vi "ConfigurationSetting_Dialog.vi"(2 "error in (no error)":errorcluster, 3 "Configuration":refnum<vi>) -> (0 "error out":errorcluster, 1 "Cancelled?":bool)   [LabVIEW 2012]
doc: "Use this template to create a dialog box with event handling."
uses:
  Config.ctl
panel:
  in  "Unblock":bool
  in  "Background WL":dbl=275.0 min=1.0 max=320.0
  in  "Knee Max":dbl min=0.0 max=40.0
  in  "Knee Min":dbl min=-40.0 max=0.0
  in  "Power Min":dbl min=0.0 max=10000.0
  in  "# Samples":i32=1 min=1 max=10
  in  "Int Time":i32=10 min=10 max=100000
  in  "Cancel":bool
  in  "Save":bool
  # "Configuration Settings"
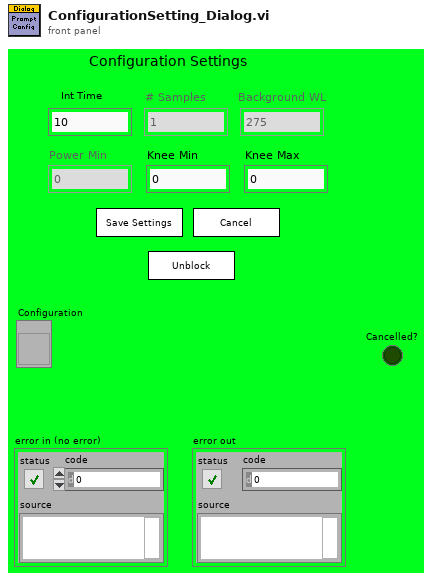
[diagram p1: front panel]
types:
  T1 = enum8{"Enabled", "Disabled", "Disabled and Grayed Out"}
  T2 = typedef "Config.ctl" = cluster{"IntTime":i32, "Samples":i32, "PowerMin":dbl, "KneeMin":dbl, "KneeMax":dbl, "BackgroundWl":dbl}
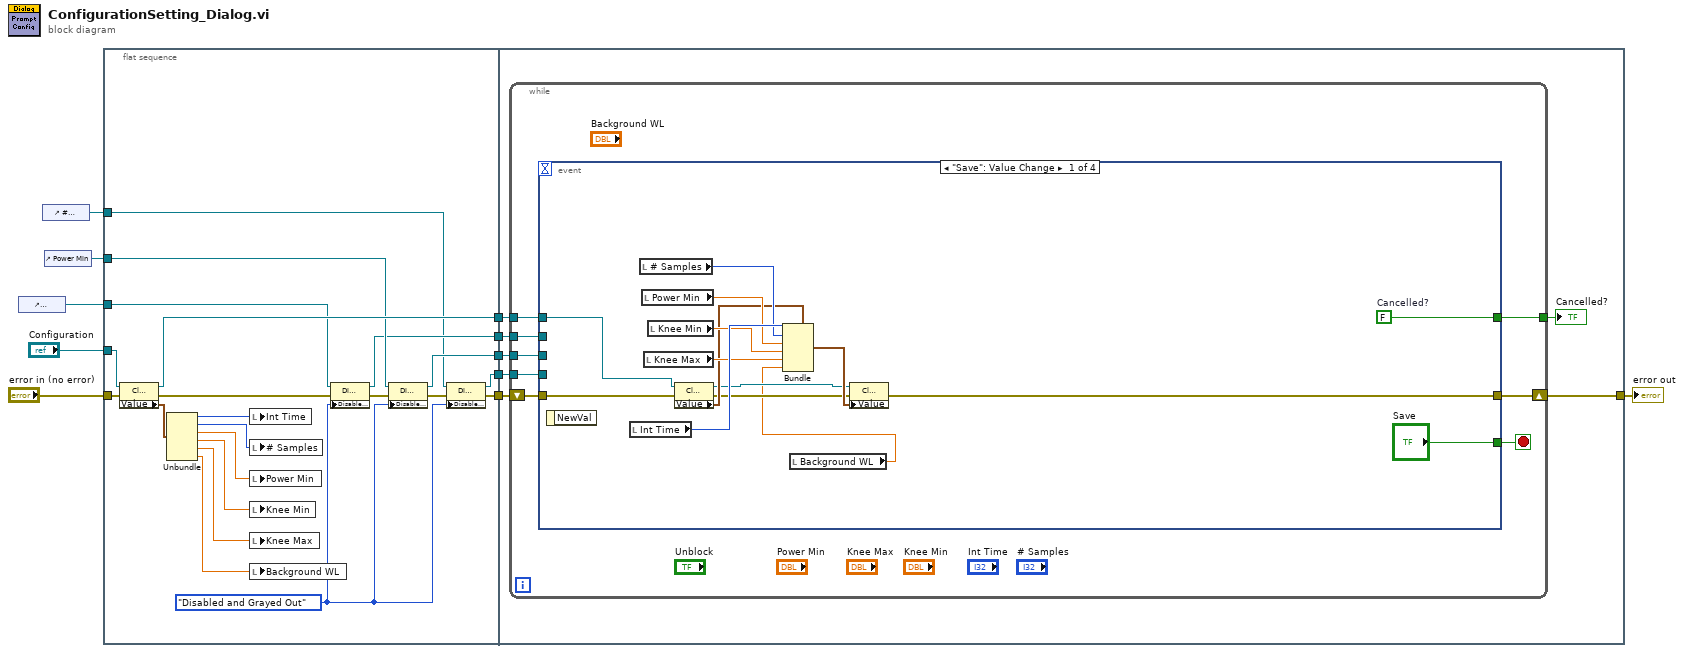
[diagram p0: block diagram]
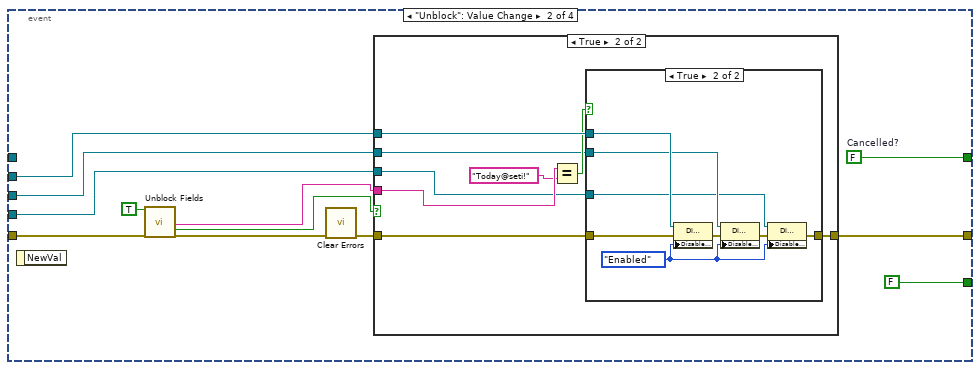
[diagram p2: hidden frame]
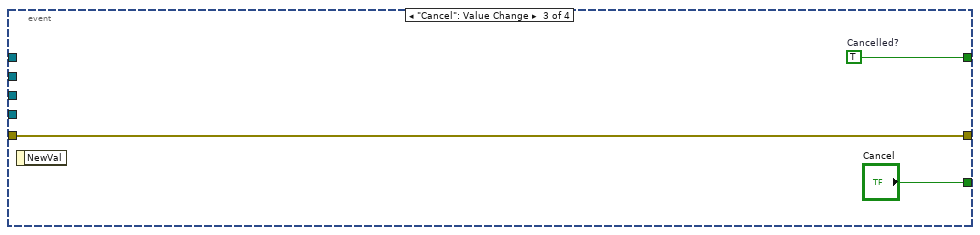
[diagram p5: hidden frame]
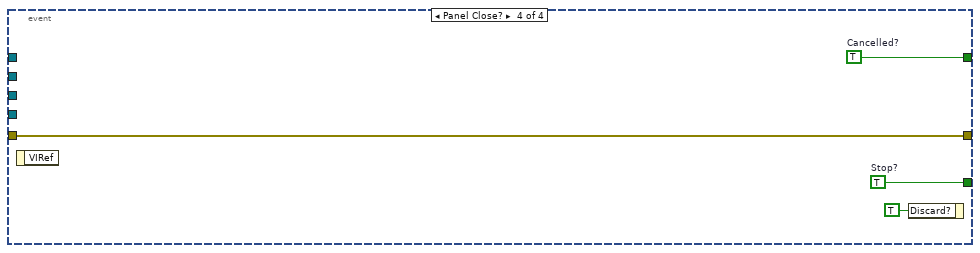
[diagram p6: hidden frame]
diagram:
  n1 = control-ref of="Background WL"() -> (w6:refnum<vi>)
  n2 = control-ref of="# Samples"() -> (w2:refnum<vi>)
  n3 = control-ref of="Power Min"() -> (w5:refnum<vi>)
  n4 = flat-sequence {
    tunnel: [w14] -> w11
    tunnel: "error in (no error)" -> [w26]
    tunnel: [w24] -> w9
    tunnel: "Configuration" -> [w27]
    tunnel: w6 -> [w20]
    tunnel: w5 -> [w19]
    tunnel: [w18] -> w4
    tunnel: [w17] -> w3
    tunnel: w2 -> [w16]
    tunnel: [w13] -> w1
    tunnel: w11 -> [w39]
    tunnel: w9 -> [w36]
    tunnel: [w38] -> w8
    tunnel: w4 -> [w35]
    tunnel: w3 -> [w34]
    tunnel: w1 -> [w33]
    frame #0 {
      w12 = T1."Disabled and Grayed Out" ("Disabled")
      n5 = property class="Clust (strict)"(reference=w27, error in=w26) -> (reference out=w24:refnum<vi>, error out=w21:errorcluster, "Value"=w25:T2)
      n6 = Unbundle(w25) -> ("IntTime"=w32:i32, "Samples"=w31:i32, "PowerMin"=w30:dbl, "KneeMin"=w29:dbl, "KneeMax"=w28:dbl, "BackgroundWl"=w23:dbl)
      n7 = local write "Int Time"(w32) -> ()
      n8 = local write "# Samples"(w31) -> ()
      n9 = local write "Power Min"(w30) -> ()
      n10 = local write "Knee Min"(w29) -> ()
      n11 = local write "Knee Max"(w28) -> ()
      n12 = local write "Background WL"(w23) -> ()
      n13 = property class="DigNum (strict)"(reference=w20, error in=w21, "DisabledEnum"=w12) -> (reference out=w18:refnum<vi>, error out=w22:errorcluster)
      n14 = property class="DigNum (strict)"(reference=w19, error in=w22, "DisabledEnum"=w12) -> (reference out=w17:refnum<vi>, error out=w15:errorcluster)
      n15 = property class="DigNum (strict)"(reference=w16, error in=w15, "DisabledEnum"=w12) -> (reference out=w13:refnum<vi>, error out=w14:errorcluster)
    }
    frame #1 {
      n16 = while {
        shift-right: [w45] -> w38
        shift-left: w39 -> [w46]
        tunnel: [w44] -> w37
        tunnel: w36 -> [w43]
        tunnel: w35 -> [w42]
        tunnel: w34 -> [w41]
        tunnel: w33 -> [w40]
        stop <- w47 stop-if-true
        n17 = event shown="[0] \"Save\": Value Change" {
          selector: _ -> [_ _ _ _]
          dyn-events: _ -> [_ _ _ _]
          timeout: _ -> [_ _ _ _]
          tunnel: ["Save" FALSE ("Stop?") "Cancel" w98] -> w47
          tunnel: [w62 w74 w95 w97] -> w44
          tunnel: w46 -> [w54 w72 w93 w96]
          tunnel: [w49 w68 w93 w96] -> w45
          tunnel: w43 -> [w55 _ _ _]
          tunnel: w42 -> [_ w67 _ _]
          tunnel: w41 -> [_ w64 _ _]
          tunnel: w40 -> [_ w63 _ _]
          event "Save": Value Change {
            w62 = FALSE  # Cancelled?
            n18 = event-data() -> ()  [unwired: 1 in, 1 out]
            n19 = local read "Int Time"() -> (w60:i32)
            n20 = local read "# Samples"() -> (w59:i32)
            n21 = local read "Power Min"() -> (w58:dbl)
            n22 = local read "Knee Max"() -> (w56:dbl)
            n23 = local read "Knee Min"() -> (w57:dbl)
            n24 = property class="Clust (strict)"(reference=w55, error in=w54) -> (reference out=w50:refnum<vi>, error out=w51:errorcluster, "Value"=w53:T2)
            n25 = local read "Background WL"() -> (w48:dbl)
            n26 = Bundle(cluster=w53, "IntTime"=w60, "Samples"=w59, "PowerMin"=w58, "KneeMin"=w57, "KneeMax"=w56, "BackgroundWl"=w48) -> (w52:T2)
            n27 = property class="Clust (strict)"(reference=w50, error in=w51, "Value"=w52) -> (error out=w49:errorcluster)  [unwired: 1 out]
          }
          event "Unblock": Value Change {
            w74 = FALSE  # Cancelled?
            n28 = event-data() -> ()  [unwired: 1 in, 1 out]
            n29 = call "Unblock Fields"("Enable"=TRUE, "error in (no error)"=w72) -> ("Password"=w65:string, "OK"=w70:bool, "error out"=w71:errorcluster)  [unwired: 15 in]
            n30 = call <vilib>:"Clear Errors.vi"("error in (no error)"=w71) -> ("error out"=w69:errorcluster)  [unwired: 6 in]
            n31 = case shown="True" w70 {
              tunnel: w69 -> [w75 w78]
              tunnel: [w75 w79] -> w68
              tunnel: w67 -> [_ w83]
              tunnel: w65 -> [_ w82]
              tunnel: w64 -> [_ w77]
              tunnel: w63 -> [_ w76]
              frame False {
              }
              frame True {
                n32 = Equal?(x=w82, y="Today@seti!") -> (x = y?=w80:bool)
                n33 = case shown="True" w80 {
                  tunnel: w83 -> [_ w91]
                  tunnel: [w84 w86] -> w79
                  tunnel: w78 -> [w84 w90]
                  tunnel: w77 -> [_ w89]
                  tunnel: w76 -> [_ w87]
                  frame False {
                  }
                  frame True {
                    w88 = T1."Enabled" ("Disabled")
                    n34 = property class="DigNum (strict)"(reference=w91, error in=w90, "DisabledEnum"=w88) -> (error out=w92:errorcluster)  [unwired: 1 out]
                    n35 = property class="DigNum (strict)"(reference=w89, error in=w92, "DisabledEnum"=w88) -> (error out=w85:errorcluster)  [unwired: 1 out]
                    n36 = property class="DigNum (strict)"(reference=w87, error in=w85, "DisabledEnum"=w88) -> (error out=w86:errorcluster)  [unwired: 1 out]
                  }
                }
              }
            }
          }
          event "Cancel": Value Change {
            w95 = TRUE  # Cancelled?
            n37 = event-data() -> ()  [unwired: 1 in, 1 out]
          }
          event Panel Close? {
            w97 = TRUE  # Cancelled?
            w98 = TRUE  # Stop?
            n38 = event-data() -> ()  [unwired: 1 in, 1 out]
            n39 = event-data("Discard?"=TRUE) -> ()  [unwired: 1 in, 1 out]
          }
        }
      }
      "Cancelled?" <- w37
    }
  }
  "error out" <- w8
